vi "CreateControllerName.vi"(9 "Device Address":i32, 11 "Model / Serial":string) -> (2 "Controller Name":string)   [LabVIEW 2012]
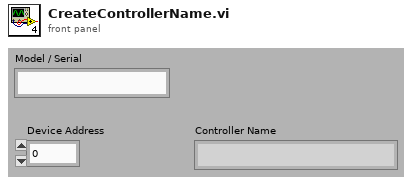
[diagram p1: front panel]
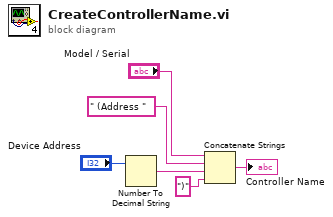
[diagram p0: block diagram]
diagram:
  n1 = Number To Decimal String(number="Device Address") -> (decimal integer string=w5:string)  [unwired: 1 in]
  n2 = Concatenate Strings("Model / Serial", " (Address " ("string"), w5, ")" ("string")) -> (→"Controller Name":string)
